vi "Start Execution.vi"(8 "error in (no error)":errorcluster, 10 "Block Instance":string, 11 "Hierarchy":string) -> (0 "error out":errorcluster)   [LabVIEW 2020, in "FlexBlocks.lvlib"]
uses:
  FlexBlocks.lvlib
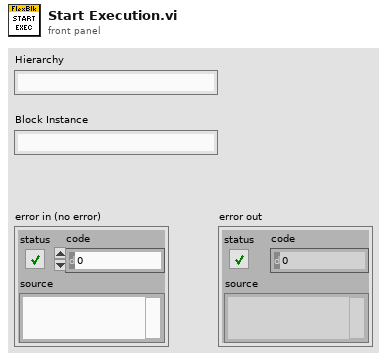
[diagram p1: front panel]
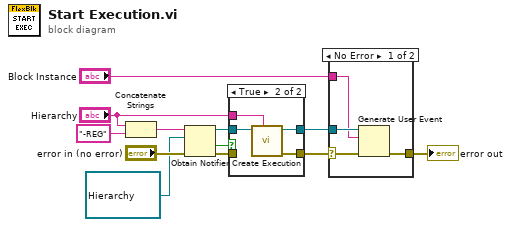
[diagram p0: block diagram]
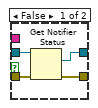
[diagram p3: hidden frame]
diagram:
  n1 = Concatenate Strings("Hierarchy", "-REG" ("string")) -> (w8:string)
  n2 = Obtain Notifier(name (unnamed)=w8, notification data type=refnum<user-event> refnum ("Reg Event"), error in (no error)="error in (no error)") -> (notifier out=w4:refnum<notifier>, created new?=w6:bool, error out=w5:errorcluster)  [unwired: 1 in]
  n3 = case shown="True" w6 {
    tunnel: w5 -> [w15 _]
    tunnel: [w14 w18] -> w9
    tunnel: [w13 w20] -> w10
    tunnel: "Hierarchy" -> [_ w19]
    tunnel: w4 -> [w16 w17]
    frame False {
      n4 = Get Notifier Status(notifier=w16, error in (no error)=w15) -> (current notification=w14:refnum<user-event>, error out=w13:errorcluster)  [unwired: 3 out]
    }
    frame True {
      n5 = call "Create Execution.vi"("Hierarchy"=w19, "Reg Notifier"=w17) -> ("error out"=w20:errorcluster, "Reg Event"=w18:refnum<user-event>)  [unwired: 8 in]
    }
  }
  n6 = case shown="No Error" w10 {
    selector: w10 -> [w22 w25]
    tunnel: w9 -> [w24 _]
    tunnel: "Block Instance" -> [w23 _]
    tunnel: [w21 w25] -> w1
    frame No Error {
      n7 = Generate User Event(user event=w24, event data cluster=w23, error in=w22) -> (error out=w21:errorcluster)  [unwired: 1 in, 1 out]
    }
    frame Error {
    }
  }
  "error out" <- w1
